vi "Increment IP Address.vi"(11 "IP Address":string) -> (1 "Unable to Increment":bool, 2 "Invalid IP Address":bool, 3 "New IP Address":string)   [LabVIEW 2020]
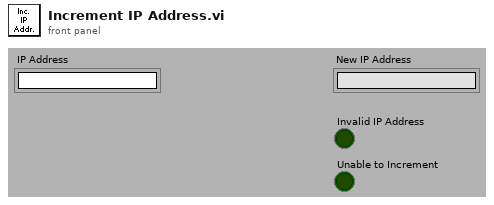
[diagram p1: front panel]
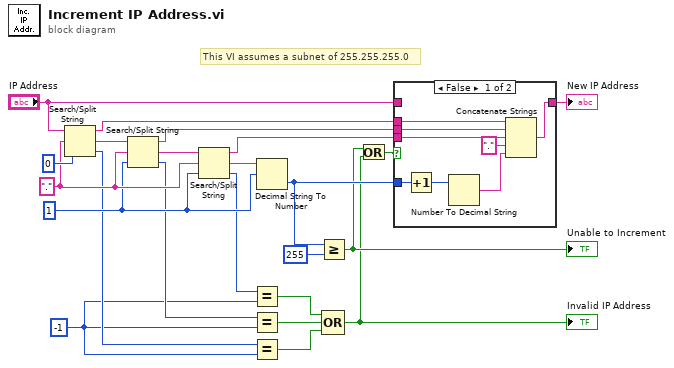
[diagram p0: block diagram]
diagram:
  w10 = -1 ("y")
  w18 = 1 ("offset (0)")
  w20 = "." ("search string/char (-)")
  # "This VI assumes a subnet of 255.255.255.0"
  n1 = Search/Split String(string="IP Address", search string/char (-)=w20, offset (0)=0) -> (substring before match=w15:string, match + rest of string=w23:string, offset of match=w13:i32)
  n2 = Search/Split String(string=w23, search string/char (-)=w20, offset (0)=w18) -> (substring before match=w16:string, match + rest of string=w21:string, offset of match=w12:i32)
  n3 = Search/Split String(string=w21, search string/char (-)=w20, offset (0)=w18) -> (substring before match=w17:string, match + rest of string=w19:string, offset of match=w11:i32)
  n4 = Equal?(x=w11, y=w10) -> (x = y?=w9:bool)
  n5 = Equal?(x=w12, y=w10) -> (x = y?=w8:bool)
  n6 = Equal?(x=w13, y=w10) -> (x = y?=w7:bool)
  n7 = Decimal String To Number(string=w19, offset=w18) -> (number=w6:i32)  [unwired: 1 in, 1 out]
  n8 = Greater Or Equal?(x=w6, y=255) -> (x >= y?=w3:bool)
  "Unable to Increment" <- w3
  n9 = Compound Arithmetic op=OR(w9, w8, w7) -> (w1:bool)
  "Invalid IP Address" <- w1
  n10 = Or(x=w3, y=w1) -> (x .or. y?=w2:bool)
  n11 = case shown="False" w2 {
    tunnel: w17 -> [w31 _]
    tunnel: w16 -> [w30 _]
    tunnel: w15 -> [w29 _]
    tunnel: [w28 w32] -> w14
    tunnel: w6 -> [w24 _]
    tunnel: "IP Address" -> [_ w32]
    frame False {
      n12 = Increment(x=w24) -> (x+1=w25:i32)
      n13 = Number To Decimal String(number=w25) -> (decimal integer string=w27:string)  [unwired: 1 in]
      n14 = Concatenate Strings(w29, w30, w31, "." ("string"), w27) -> (w28:string)
    }
    frame True {
    }
  }
  "New IP Address" <- w14
